vi "Configure Clock Delay.vi"(7 "Clock Delay Resolution (1E-8 s)":dbl=1e-08 format="%.8e", 8 "error in (no error)":errorcluster, 9 "Clock Time Delay (2.67E-8 s)":dbl=2.67e-08 format="%.8e", 10 "Enable Clock Delay (F: Disable)":bool, 11 "VISA resource name":refnum<visa-resource-name>) -> (0 "error out":errorcluster, 3 "VISA resource name out":refnum<visa-resource-name>)   [LabVIEW 2018, in "Agilent PSG MXG Series.lvlib"]
doc: "Configures the clock signal delay function.\n\n<b>Note:</b>\nIt is applicable for N5172B/82B with <b>Option UN7</b> only."
uses:
  Agilent PSG MXG Series.lvlib
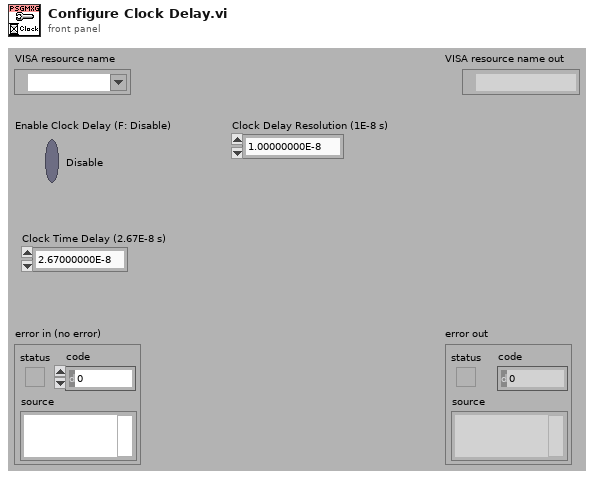
[diagram p1: front panel]
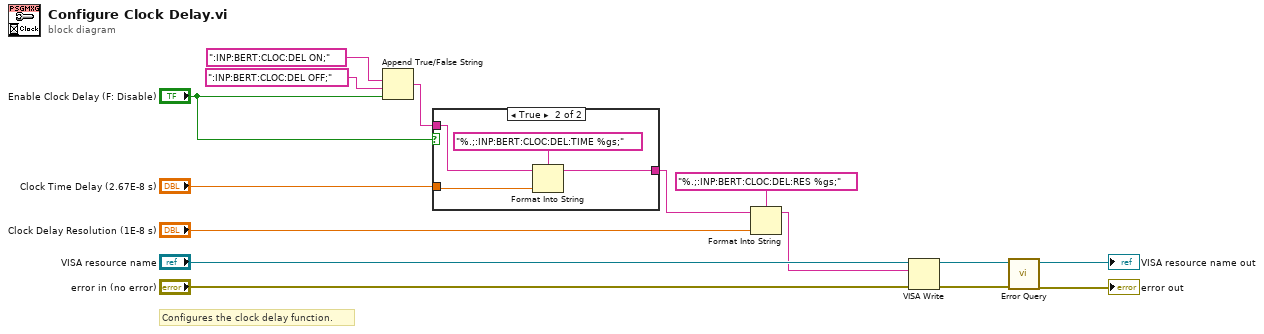
[diagram p0: block diagram]
diagram:
  # "Configures the clock delay function."
  n1 = Append True/False String(1:"Enable Clock Delay (F: Disable)", 2:":INP:BERT:CLOC:DEL OFF;", 3:":INP:BERT:CLOC:DEL ON;") -> (0:w4:string)  [unwired: 1 in]
  n2 = case shown="True" "Enable Clock Delay (F: Disable)" {
    tunnel: "Clock Time Delay (2.67E-8 s)" -> [_ w20]
    tunnel: [w16 w19] -> w5
    tunnel: w4 -> [w16 w17]
    frame False {
    }
    frame True {
      n3 = Format Into String(format string="%.;:INP:BERT:CLOC:DEL:TIME %gs;", initial string=w17, w20) -> (resulting string=w19:string)  [unwired: 1 in, 1 out]
    }
  }
  n4 = Format Into String(format string="%.;:INP:BERT:CLOC:DEL:RES %gs;", initial string=w5, "Clock Delay Resolution (1E-8 s)") -> (resulting string=w8:string)  [unwired: 1 in, 1 out]
  n5 = VISA Write(VISA resource name="VISA resource name", write buffer=w8, error in (no error)="error in (no error)") -> (VISA resource name out=w13:refnum<visa-resource-name>, error out=w12:errorcluster)  [unwired: 1 out]
  n6 = call "Error Query.vi"("error in (no error)"=w12, "VISA resource name"=w13) -> ("error out"=→"error out":errorcluster, "VISA resource name out"=→"VISA resource name out":refnum<visa-resource-name>)  [unwired: 6 in, 2 out]
